vi "Write Base I32.vi"(5 "timestamps":timestamp[](array[numeric]), 7 "index_channel":u32, 8 "error in":errorcluster, 9 "data":i32[][](array[numeric]), 10 "channels":u32[](array[numeric]), 11 "Writer":refnum<class "Synnax Writer.lvclass">) -> (0 "error out":errorcluster, 3 "Writer Out":refnum<class "Synnax Writer.lvclass">)   [LabVIEW 2026, in "synnax_clib.lvlib" / "Synnax Writer.lvclass"]
doc: "SYNNAX_EXPORT int32_t synnax_writer_write(\n SynnaxWriter writer,\n uint32_t channel,\n const double *data,\n uint64_t sample_count,\n SynnaxError err\n);"
uses:
  Synnax Writer.lvclass
  Synnax Writer.lvclass/Synnax Writer.ctl
  synnax_clib.lvlib
  synnax_clib.dll
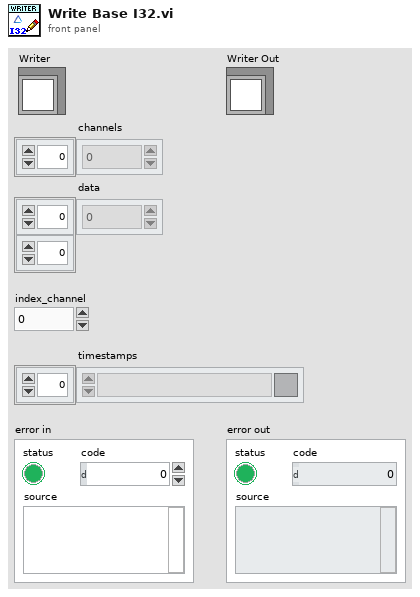
[diagram p1: front panel]
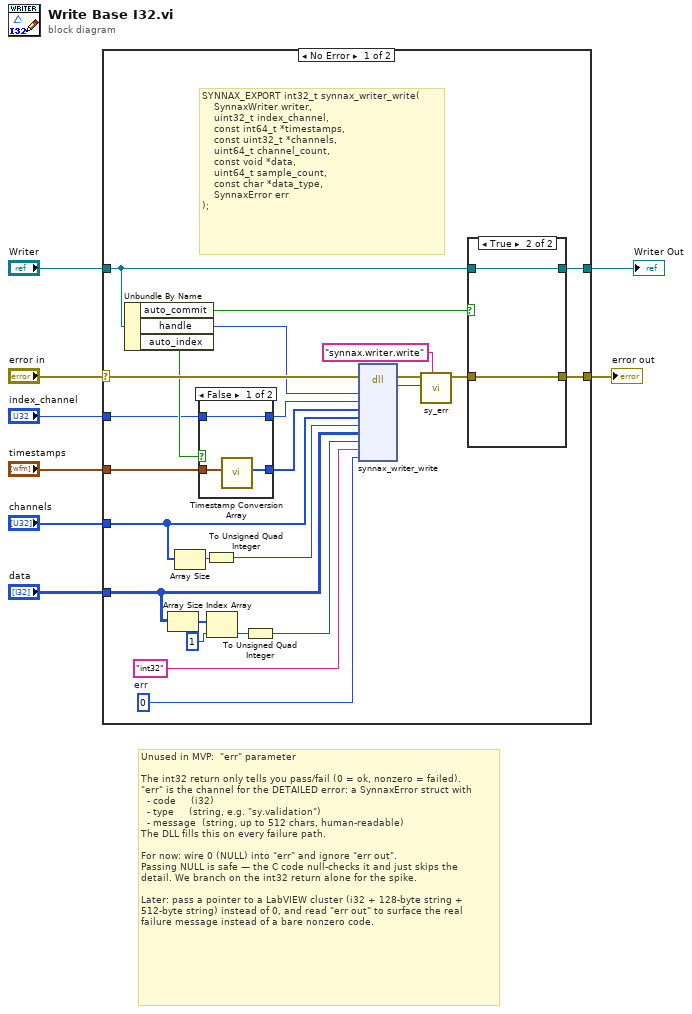
[diagram p0: block diagram]
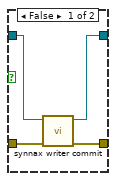
[diagram p2: hidden frame]
diagram:
  # "Unused in MVP:  \"err\" parameter\n\nThe int32 return only tells you pass/fail (0 = ok, nonzero = failed).\n\"err\" is the channel for the DETAILED error: a SynnaxError struct with\n  - code     (i32)\n  - type     (string, e.g. \"sy.validation\")\n  - message  (string, up to 512 chars, human-readable)\nThe DLL fills this on every failure path.\n\nFor now: wire 0 (NULL) into \"err\" and ignore \"err out\".\nPassing NULL is safe — the C code null-checks it and just skips the\ndetail. We branch on the int32 return alone for the spike.\n\nLater: pass a pointer to a LabVIEW cluster (i32 + 128-byte string +\n512-byte string) instead of 0, and read \"err out\" to surface the real\nfailure message instead of a bare nonzero code."
  n1 = case shown="No Error" "error in" {
    selector: "error in" -> [w22 w44]
    tunnel: "index_channel" -> [w17 _]
    tunnel: [w14 w44] -> w7
    tunnel: "channels" -> [w28 _]
    tunnel: "data" -> [w26 _]
    tunnel: "timestamps" -> [w20 _]
    tunnel: "Writer" -> [w12 w43]
    tunnel: [w13 w43] -> w1
    frame No Error {
      w9 = u64 0  # err
      # "SYNNAX_EXPORT int32_t synnax_writer_write(\n    SynnaxWriter writer,\n    uint32_t index_channel,\n    const int64_t *timestamps,\n    const uint32_t *channels,\n    uint64_t channel_count,\n    const void *data,\n    uint64_t sample_count,\n    const char *data_type,\n    SynnaxError err\n);"
      n2 = Unbundle By Name(w12) -> ("auto_commit"=w11:bool, "handle"=w21:u64, "auto_index"=w18:bool)
      n3 = Array Size(array=w26) -> (size(s)=w25:i32[])
      n4 = Array Size(array=w28) -> (size(s)=w30:i32)
      n5 = case shown="False" w18 {
        tunnel: w20 -> [w42 _]
        tunnel: [w41 _] -> w19
        tunnel: [w40 _] -> w16
        tunnel: w17 -> [w40 _]
        frame False {
          n6 = call "Timestamp Conversion Array.vi"("timestamps"=w42) -> ("timestamps (ns)"=w41:i64[])  [unwired: 9 in]
        }
        frame True {
        }
      }
      n7 = To Unsigned Quad Integer(1:w30) -> (0:w29:u64)
      n8 = Index Array(array=w25, index=1) -> (element=w24:i32)
      n9 = To Unsigned Quad Integer(1:w24) -> (0:w27:u64)
      n10 = dll-call lib="C/synnax/client/labview/synnax_clib.*" fn="synnax_writer_write"(error in=w22, "writer"=w21, "index_channel"=w16, "timestamps"=w19, "channels"=w28, "channel_count"=w29, "data"=w26, "sample_count"=w27, "data_type"="int32", "err"=w9) -> (error out=w33:errorcluster, "return type"=w32:i32)  [unwired: 11 in, 1 out]
      n11 = call "sy_err.vi"("source"="synnax.writer.write", "error code"=w32, "error in (no error)"=w33) -> ("error out"=w15:errorcluster)  [unwired: 8 in]
      n12 = case shown="True" w11 {
        tunnel: w15 -> [w37 w38]
        tunnel: [w36 w38] -> w14
        tunnel: w12 -> [w35 w39]
        tunnel: [w34 w39] -> w13
        frame False {
          n13 = call "synnax writer commit.vi"("error in"=w37, "Writer"=w35) -> ("error out"=w36:errorcluster, "Writer Out"=w34:refnum<class "Synnax Writer.lvclass">)  [unwired: 7 in, 1 out]
        }
        frame True {
        }
      }
    }
    frame Error {
    }
  }
  "error out" <- w7
  "Writer Out" <- w1
